vi "Read InstrumentCommunication.vi"(8 "error in (no error)":errorcluster, 11 "InstrumentCommunication in":refnum<class "InstrumentCommunication.lvclass">) -> (0 "error out":errorcluster, 2 "InstrumentCommunication":string[][](array[string]), 3 "InstrumentCommunication out":refnum<class "InstrumentCommunication.lvclass">)   [LabVIEW 2019, in "HardwareSetup_model001.lvlib" / "InstrumentCommunication.lvclass"]
uses:
  InstrumentCommunication.lvclass
  InstrumentCommunication.lvclass/InstrumentCommunication.ctl
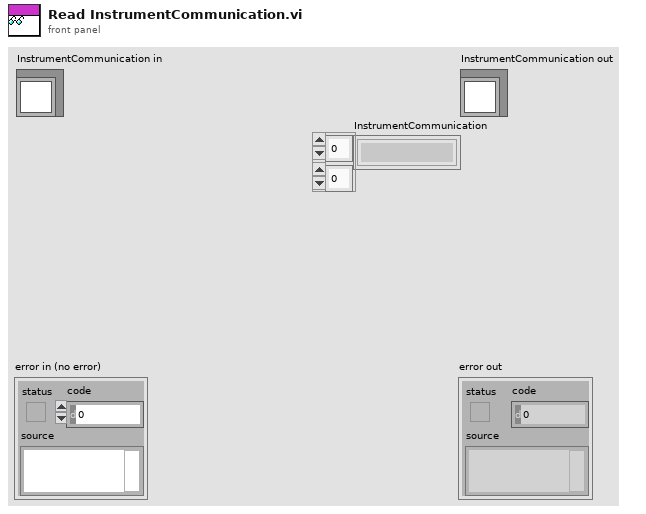
[diagram p1: front panel]
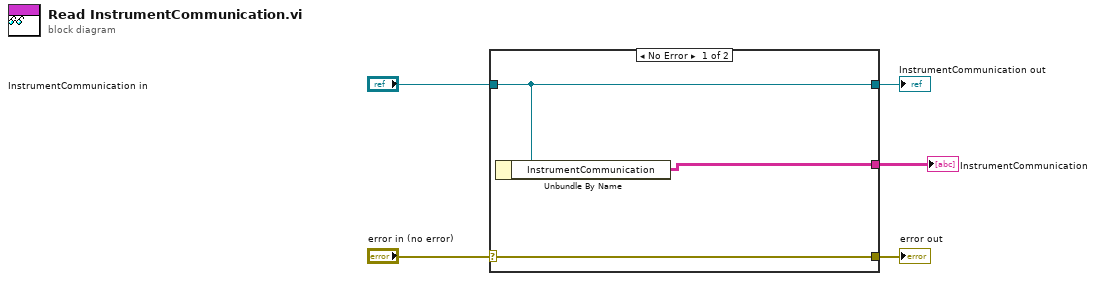
[diagram p0: block diagram]
diagram:
  n1 = case shown="No Error" "error in (no error)" {
    selector: "error in (no error)" -> [w8 w9]
    tunnel: [w8 w9] -> w4
    tunnel: [w7 w10] -> w2
    tunnel: "InstrumentCommunication in" -> [w7 w10]
    tunnel: [w6 _] -> w1
    frame No Error {
      n2 = Unbundle By Name(w7) -> ("InstrumentCommunication"=w6:string[][])
    }
    frame Error {
    }
  }
  "error out" <- w4
  "InstrumentCommunication out" <- w2
  "InstrumentCommunication" <- w1
